vi "WLAN - RxMeasure - DLL - VI.vi"() -> ()   [LabVIEW 2012]
uses:
  TV/RW/Includes/WLAN - TV - OPPO - RW - INC - TV_Rx_Measurements.ctl
  TV/RW/Includes/WLAN - NIStandardDefine.ctl
panel:
  in  "GenWvfmName":string
  in  "Path Loss":dbl
  in  "RxPower":dbl
  in  "RF:Frequency (Hz)":dbl
  out "error out 3":errorcluster
  out "error out 2":errorcluster
  out "error out":errorcluster
  in  "Rx Measurements Settings":T1={"Channel Bandwidth (Hz)"=4.0, "Idle Interval (s)"=40000000.0, "MCS Index"=0, "80211n PLCP Frame Format"=0, "Payload Data Length (bytes)"=0, "OFDM Data Rate (Mbps)"=1024, "DSSS Data Rate (Mbps)"=0, "#N_SS"=0, "NIStandard"=enum."80211A/G/J/P(OFDM)"} {"DSSS Data Rate (Mbps)" items=["1", "2", "5.5 CCK", "5.5 PBCC", "11 CCK", "11 PBCC", "22", "33"]; "OFDM Data Rate (Mbps)" items=["6", "9", "12", "18", "24", "36", "48", "54"]; "80211n PLCP Frame Format" items=["Mixed Format", "Greenfield Format"]}
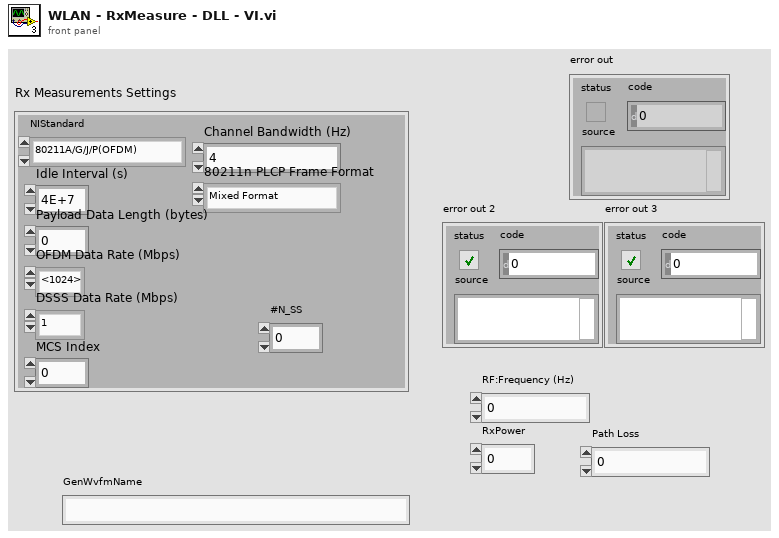
[diagram p1: front panel]
types:
  T1 = typedef "WLAN - TV - OPPO - RW - INC - TV_Rx_Measurements.ctl" = cluster{"Channel Bandwidth (Hz)":dbl, "Idle Interval (s)":dbl, "MCS Index":i32, "80211n PLCP Frame Format":i32, "Payload Data Length (bytes)":i32, "OFDM Data Rate (Mbps)":i32, "DSSS Data Rate (Mbps)":i32, "#N_SS":i32, "NIStandard":T2}
  T2 = typedef "WLAN - NIStandardDefine.ctl" = enum32{"80211A/G/J/P(OFDM)", "80211B/G(DSSS)", "80211GDSSSOFDM", "80211NMIMOOFDM", "80211ACMIMOOFDM"}
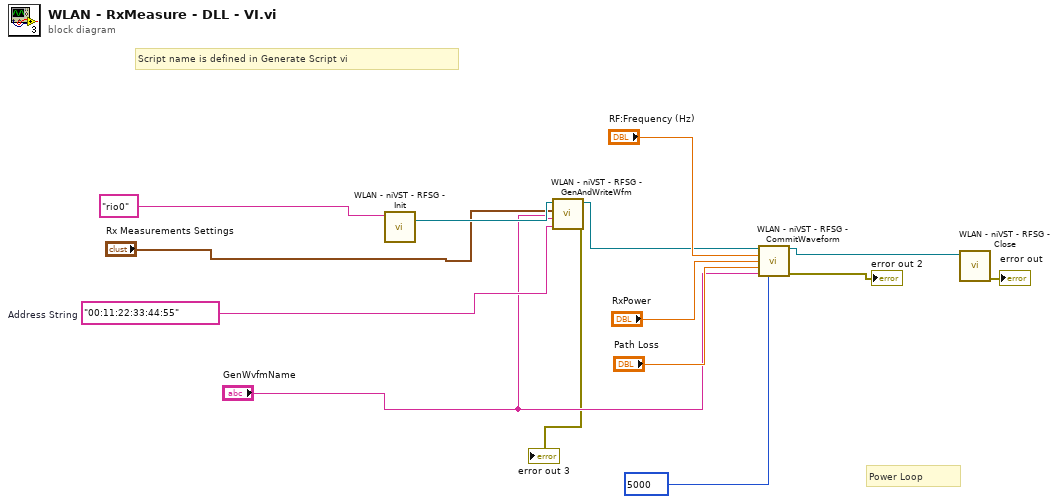
[diagram p0: block diagram]
diagram:
  w4 = "00:11:22:33:44:55"  # Address String
  # "Power Loop"
  # "Script name is defined in Generate Script vi"
  n1 = call "WLAN - niVST - RFSG - Init.vi"("RFSG Handle"="rio0") -> ("RFSG handle out"=w6:refnum<k15>)  [unwired: 9 in, 1 out]
  n2 = call "WLAN - niVST - RFSG - GenAndWriteWfm.vi"("Address String"=w4, "WaveformNamePostfix"="GenWvfmName", "Rx Measurements Settings"="Rx Measurements Settings", "instrument handle"=w6) -> ("error out"=→"error out 3":errorcluster, "RFSG out"=w2:refnum<k15>)  [unwired: 6 in]
  n3 = call "WLAN - niVST - RFSG - CommitWaveform.vi"("RFSG handle"=w2, "RF:Frequency (Hz)"="RF:Frequency (Hz)", "RxPower"="RxPower", "Path Loss"="Path Loss", "WvformNamePostfixed"="GenWvfmName", "Number of Packets"=5000) -> ("RFSG handle out"=w8:refnum<k15>, "error out"=→"error out 2":errorcluster)  [unwired: 8 in]
  n4 = call "WLAN - niVST - RFSG - Close.vi"("RFSG handle"=w8) -> ("error out"=→"error out":errorcluster)  [unwired: 10 in]
